vi "generate array.vi"(11 "json strings":string[](array[string])) -> (3 "array string":string)   [LabVIEW 2013, in "json generator.lvlib"]
uses:
  json generator.lvlib
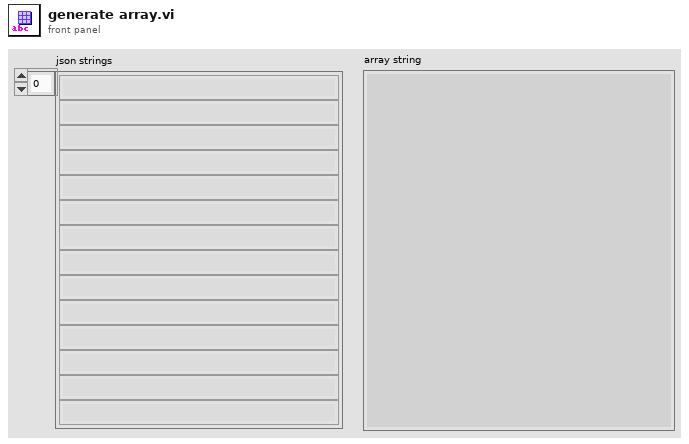
[diagram p1: front panel]
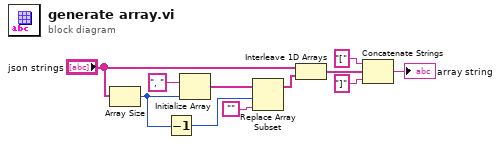
[diagram p0: block diagram]
diagram:
  n1 = Array Size(array="json strings") -> (size(s)=w3:i32)
  n2 = Decrement(x=w3) -> (x-1=w2:i32)
  n3 = Initialize Array(", ", w3) -> (w10:string[])
  n4 = Replace Array Subset(array=w10, new element="", index=w2) -> (w4:string[])
  n5 = Interleave 1D Arrays("json strings", w4) -> (w8:string[])
  n6 = Concatenate Strings("[" ("string"), w8, "]" ("string")) -> (→"array string":string)
